vi "Angle to Encoder Ticks.vi"(4 "Length/Tick":dbl, 6 "Triangle Angle(degrees)":dbl, 8 "Distance from Pivot Point to Arm Mount(in)":dbl, 9 "Distance from Pivot Point to Drive Mount(in)":dbl, 10 "Minimum Linear Actuator Length":dbl, 11 "Angle(degrees)":dbl) -> (2 "Encoder Ticks":dbl)   [LabVIEW 2015]
panel:
  # "These controls will be replaced with constants when the robot is built."
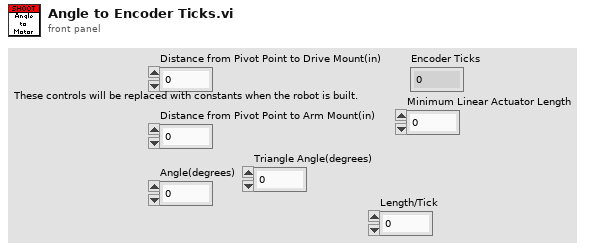
[diagram p1: front panel]
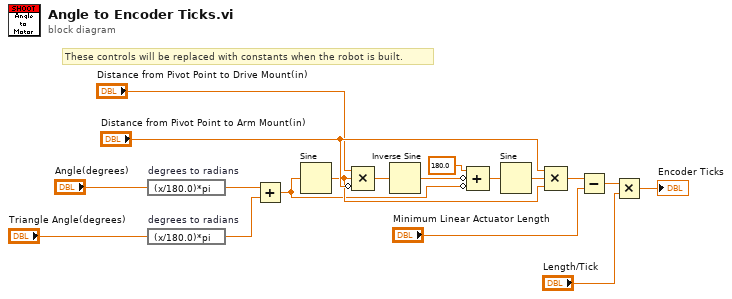
[diagram p0: block diagram]
diagram:
  # "These controls will be replaced with constants when the robot is built."
  n1 = expression code="(x/180.0)*pi" "degrees to radians"("Angle(degrees)") -> (w2:dbl)
  n2 = expression code="(x/180.0)*pi" "degrees to radians"("Triangle Angle(degrees)") -> (w1:dbl)
  n3 = Add(x=w2, y=w1) -> (x+y=w5:dbl)
  n4 = Sine(x=w5) -> (sin(x)=w15:dbl)
  n5 = Compound Arithmetic op=MULTIPLY("Distance from Pivot Point to Drive Mount(in)", w15, invert "Distance from Pivot Point to Arm Mount(in)") -> (w17:dbl)
  n6 = Inverse Sine(1:w17) -> (0:w13:dbl)
  n7 = Compound Arithmetic op=ADD(180.0 ("value"), invert w13, invert w5) -> (w16:dbl)
  n8 = Sine(x=w16) -> (sin(x)=w11:dbl)
  n9 = Compound Arithmetic op=MULTIPLY("Distance from Pivot Point to Arm Mount(in)", w11, w15) -> (w7:dbl)
  n10 = Subtract(x=w7, y="Minimum Linear Actuator Length") -> (x-y=w8:dbl)
  n11 = Multiply(x=w8, y="Length/Tick") -> (x*y=→"Encoder Ticks":dbl)
